vi "Store Errors.vi"(1 "New Error":string) -> ()   [LabVIEW 2019]
panel:
  out "Strings with Errors":string[](array[string])
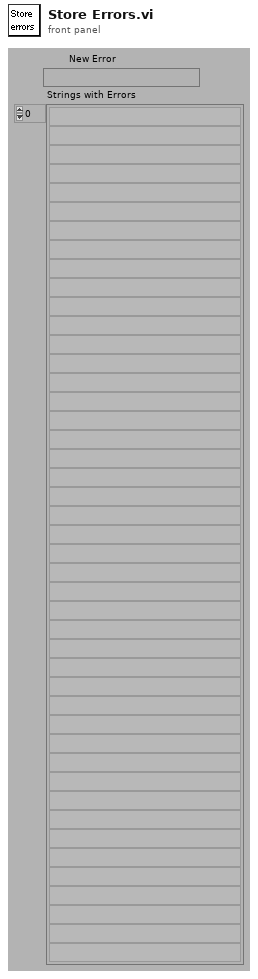
[diagram p1: front panel]
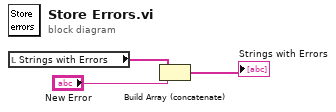
[diagram p0: block diagram]
diagram:
  n1 = local read "Strings with Errors"() -> (w3:string[])
  n2 = Build Array (concatenate)(w3, "New Error") -> (→"Strings with Errors":string[])
